vi "Configure Bus Definition.vi"   [LabVIEW 2016, in "Agilent 2000 3000 X-Series.lvlib"]
doc: "Configures bus definition."
uses:
  Agilent 2000 3000 X-Series.lvlib
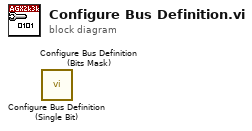
[diagram p0: block diagram]
diagram:
  n1 = call "Configure Bus Definition (Single Bit).vi"() -> ()  [unwired: 10 in, 2 out]
  n2 = call "Configure Bus Definition (Bits Mask).vi"() -> ()  [unwired: 10 in, 2 out]
